vi "串口实验11.vi"() -> ()   [LabVIEW 2018]
uses:
  <vilib>/Instr/_visa.llb/VISA Configure Serial Port (Instr).vi
panel:
  out "航向（度）":sgl
  out "速度（节）":dbl
  out "经度方向":string
  out "经度":i32
  out "经分":dbl
  out "read buffer":string
  out "分":i32
  out "秒":dbl
  out "时":i32
  out "纬度方向":string
  out "纬分":dbl
  out "纬度":i32
  out "定位成功":bool
  out "读取缓冲区":string
  out "RMC":bool
  out "第一个子数组":u8[](array[numeric])
  in  "baud rate (9600)":u32=9600 caption="波特率(9600)"
  in  "VISA resource name":refnum<visa-resource-name> caption="VISA资源名称"
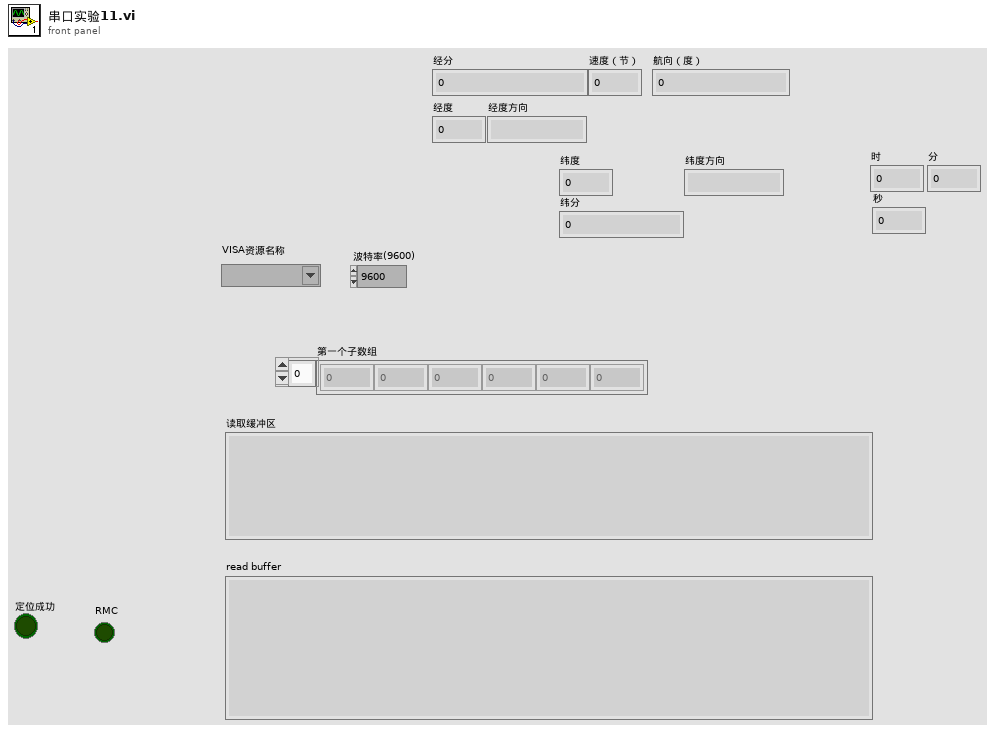
[diagram p1: front panel]
types:
  T1 = cluster{"[0]":u8, "[1]":u8, "[2]":u8, "[3]":u8, "[4]":u8, "[5]":u8, "[6]":u8, "[7]":u8, "[8]":u8}
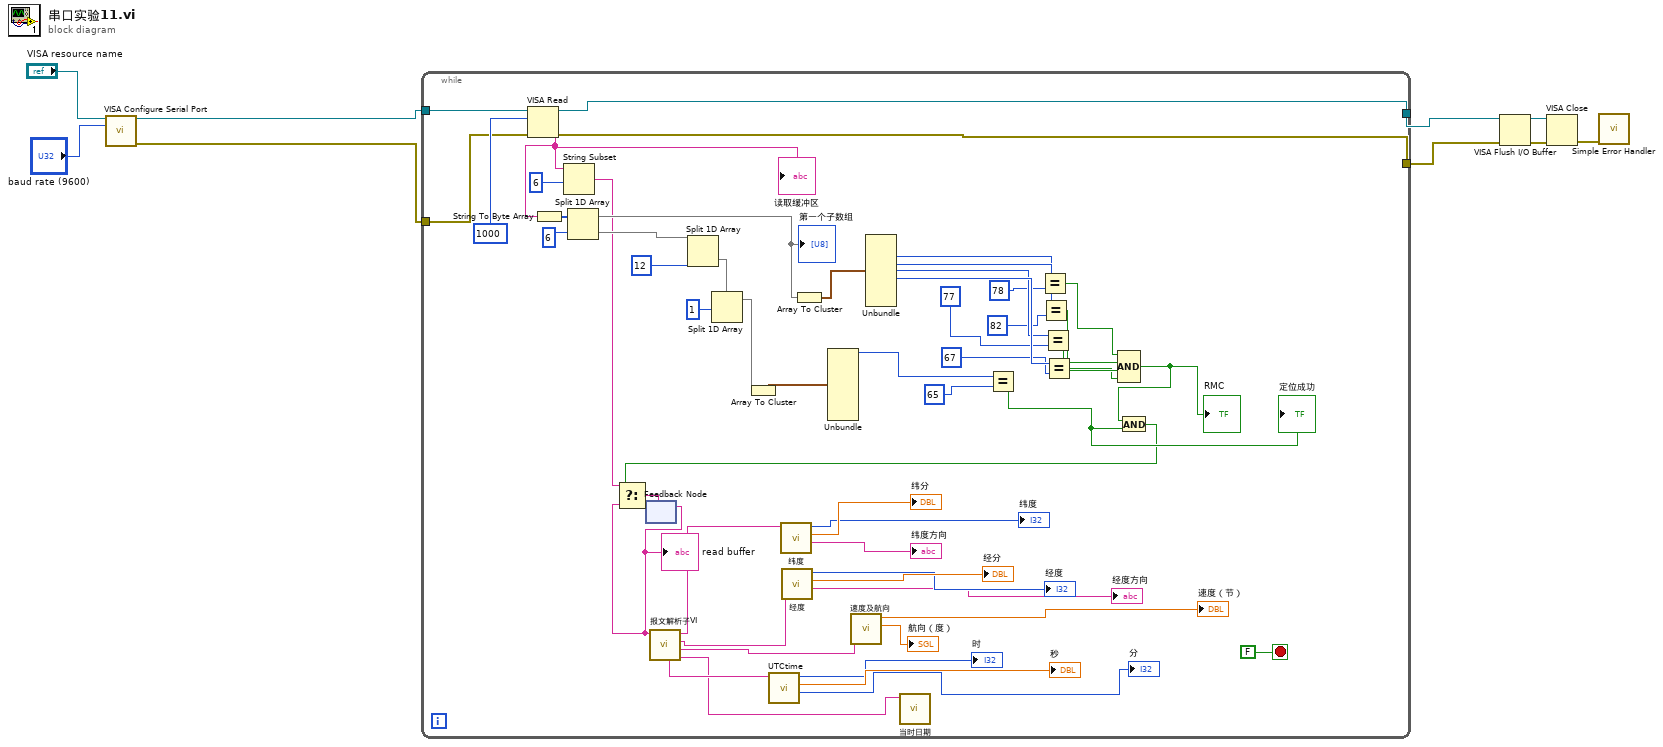
[diagram p0: block diagram]
diagram:
  n1 = call-poly "VISA Configure Serial Port"("VISA resource name"="VISA resource name", "baud rate (9600)"="baud rate (9600)") -> ("VISA resource name out"=w2:refnum<visa-resource-name>, "error out"=w1:errorcluster)  [unwired: 12 in]
  n2 = while {
    tunnel: w2 -> [w35]
    tunnel: w1 -> [w34]
    tunnel: [w33] -> w6
    tunnel: [w32] -> w5
    stop <- FALSE stop-if-true
    n3 = VISA Read(VISA resource name=w35, byte count=u32 1000 ("字节总数"), error in (no error)=w34) -> (VISA resource name out=w33:refnum<visa-resource-name>, read buffer=w61:string, error out=w32:errorcluster)  [unwired: 1 out]
    "读取缓冲区" <- w61
    n4 = String To Byte Array(string=w61) -> (unsigned byte array=w60:u8[])
    n5 = String Subset(string=w61, offset (0)=6 ("偏移量(0)")) -> (substring=w19:string)  [unwired: 1 in]
    n6 = Split 1D Array(array=w60, index=6 ("索引")) -> (first subarray=w58:u8[], second subarray=w31:u8[])
    "第一个子数组" <- w58
    n7 = feedback #1() -> (w17:string)  [unwired: 1 in]
    "read buffer" <- w17
    n8 = call "报文解析子VI.vi"("剔除报文标识字符串"=w17) -> ("当时日期"=w16:string, "速度及航向"=w23:string, "经度"=w21:string, "纬度"=w22:string, "UTCtime"=w24:string)  [unwired: 6 in]
    n9 = Split 1D Array(array=w31, index=12 ("索引")) -> (second subarray=w51:u8[])  [unwired: 1 out]
    n10 = Split 1D Array(array=w51, index=1 ("索引")) -> (first subarray=w41:u8[])  [unwired: 1 out]
    n11 = Array To Cluster(array=w41) -> (cluster=w40:T1)
    n12 = call "UTCtime.vi"("UTCtime输入"=w24) -> ("分"=→"分":i32, "秒"=→"秒":dbl, "时"=→"时":i32)  [unwired: 8 in]
    n13 = call "纬度.vi"("纬度"=w22) -> ("纬度方向"=→"纬度方向":string, "纬分"=→"纬分":dbl, "纬度"=→"纬度":i32)  [unwired: 8 in]
    n14 = call "经度.vi"("经度"=w21) -> ("经度方向"=→"经度方向":string, "经分"=→"经分":dbl, "经度"=→"经度":i32)  [unwired: 8 in]
    n15 = Array To Cluster(array=w58) -> (cluster=w57:T1)
    n16 = Unbundle(w40) -> ("[0]"=w39:u8)  [unwired: 8 out]
    n17 = call "速度及航向.vi"("速度及航向输入"=w23) -> ("航向（度）"=→"航向（度）":sgl, "速度（节）"=→"速度（节）":dbl)  [unwired: 9 in]
    n18 = Unbundle(w57) -> ("[2]"=w48:u8, "[3]"=w49:u8, "[4]"=w55:u8, "[5]"=w56:u8)  [unwired: 5 out]
    n19 = call "当时日期.vi"("待处理日期"=w16) -> ()  [unwired: 8 in, 3 out]
    n20 = Equal?(x=w39, y=u8 65) -> (x = y?=w36:bool)
    "定位成功" <- w36
    n21 = Equal?(x=w48, y=u8 78) -> (x = y?=w45:bool)
    n22 = Equal?(x=w49, y=u8 82) -> (x = y?=w44:bool)
    n23 = Equal?(x=w55, y=u8 77) -> (x = y?=w43:bool)
    n24 = Equal?(x=w56, y=u8 67) -> (x = y?=w42:bool)
    n25 = Compound Arithmetic op=AND ("复合运算")(w45, w44, w43, w42) -> (w37:bool)
    "RMC" <- w37
    n26 = And(x=w37, y=w36) -> (x .and. y?=w20:bool)
    n27 = Select(t=w19, s=w20, f=w17) -> (s? t:f=w18:string)
    n28 = feedback-in #1(w18) -> ()
  }
  n29 = VISA Flush I/O Buffer(VISA resource name=w6, error in (no error)=w5) -> (VISA resource name out=w9:refnum<visa-resource-name>, error out=w8:errorcluster)  [unwired: 1 in]
  n30 = VISA Close(VISA resource name=w9, error in (no error)=w8) -> (error out=w7:errorcluster)
  n31 = call <vilib>:"Simple Error Handler.vi"("error in (no error)"=w7) -> ()  [unwired: 4 in, 5 out]
